vi "Avantes - AVS_GetScopeData.vi"(8 "error in (no error)":errorcluster, 10 "a_pTimeLabel":u32, 11 "AVS Settings In":T1) -> (0 "error out":errorcluster, 1 "a_pSpectrum":dbl[](array[numeric]), 2 "a_pTimeLabel 2":u32, 3 "AVS Settings Out":T1)   [LabVIEW 2014, in "AvaSpec.lvlib" / "Avantes Spectrometer Functions.lvlib"]
doc: "Grab intensity values for all pixels"
uses:
  Avantes Spectrometer Functions.lvlib
  AVS settings.ctl
  AvaSpec.lvlib
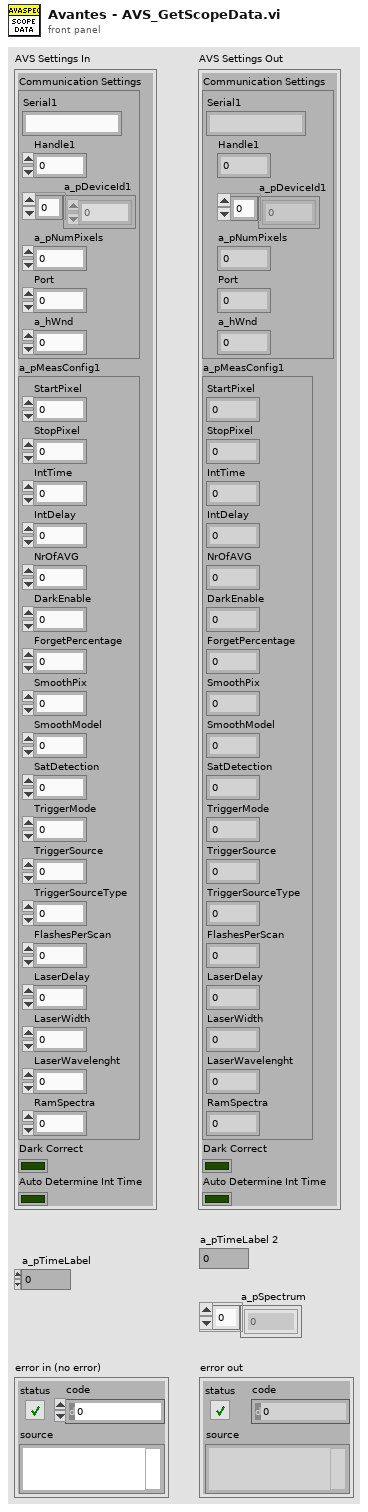
[diagram p1: front panel]
types:
  T1 = typedef "AvaSpec.lvlib/AVS settings.ctl" = cluster{"Communication Settings":cluster{"Serial1":string, "Handle1":i32, "a_pDeviceId1":u8[], "a_pNumPixels":u16, "Port":i32, "a_hWnd":i32}, "a_pMeasConfig1":cluster{"StartPixel":u16, "StopPixel":u16, "IntTime":sgl, "IntDelay":u32, "NrOfAVG":u32, "DarkEnable":u8, "ForgetPercentage":u8, "SmoothPix":u16, "SmoothModel":u8, "SatDetection":u8, "TriggerMode":u8, "TriggerSource":u8, "TriggerSourceType":u8, "FlashesPerScan":u16, "LaserDelay":u32, "LaserWidth":u32, "LaserWavelenght":sgl, "RamSpectra":u16}, "Dark Correct":bool, "Auto Determine Int Time":bool}
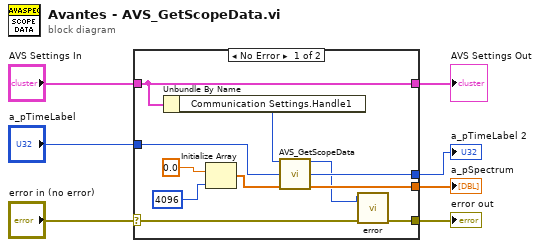
[diagram p0: block diagram]
diagram:
  n1 = case shown="No Error" "error in (no error)" {
    selector: "error in (no error)" -> [w9 w20]
    tunnel: [w12 w19] -> w1
    tunnel: "AVS Settings In" -> [w12 w19]
    tunnel: "a_pTimeLabel" -> [w14 _]
    tunnel: [w10 w20] -> w6
    tunnel: [w13 _] -> w4
    tunnel: [w11 _] -> w3
    frame No Error {
      n2 = Unbundle By Name(w12) -> ("Communication Settings.Handle1"=w18:i32)
      n3 = Initialize Array(0.0 ("element"), 4096 ("dimension size")) -> (w15:dbl[])
      n4 = call "AVS_GetScopeData.vi"("a_hDevice"=w18, "a_pTimeLabel"=w14, "a_pSpectrum"=w15) -> ("Output Value"=w8:i32, "a_pTimeLabel"=w11:u32, "a_pSpectrum"=w13:dbl[])  [unwired: 10 in]
      n5 = call "error.vi"("error in (no error)"=w9, "Output Value"=w8) -> ("error out"=w10:errorcluster)  [unwired: 9 in]
    }
    frame Error {
    }
  }
  "error out" <- w6
  "a_pSpectrum" <- w4
  "a_pTimeLabel 2" <- w3
  "AVS Settings Out" <- w1
